vi "DecodeRatio.vi"(1 "Data In":u8[](array[numeric])) -> (0 "Data Out":dbl[](array[numeric]))   [LabVIEW 2014, in "navX-MXP IMU.lvlib"]
uses:
  navX-MXP IMU.lvlib
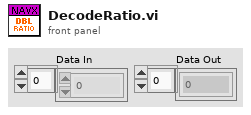
[diagram p1: front panel]
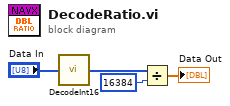
[diagram p0: block diagram]
diagram:
  n1 = call "DecodeInt16.vi"("Data In"="Data In") -> ("Data Out"=w2:i16[])
  n2 = Divide(x=w2, y=16384) -> (x/y=→"Data Out":dbl[])
